vi "AlarmEngineBuildTags.vi"(8 "error in (no error)":errorcluster, 10 "Config":T2, 11 "ModuleID":string) -> (0 "error out":errorcluster, 3 "Tag Refs":T1)   [LabVIEW 2020, in "AlarmEngine.lvlib"]
uses:
  AlarmEngine.lvlib
  3621d97f-605c-4e6f-807d-a17beb1ed3ae.vi
  f8fd6500-b03e-4021-a7cb-1885c161f361.vi
  <vilib>/Tag Engine/Tag/Tag.lvclass
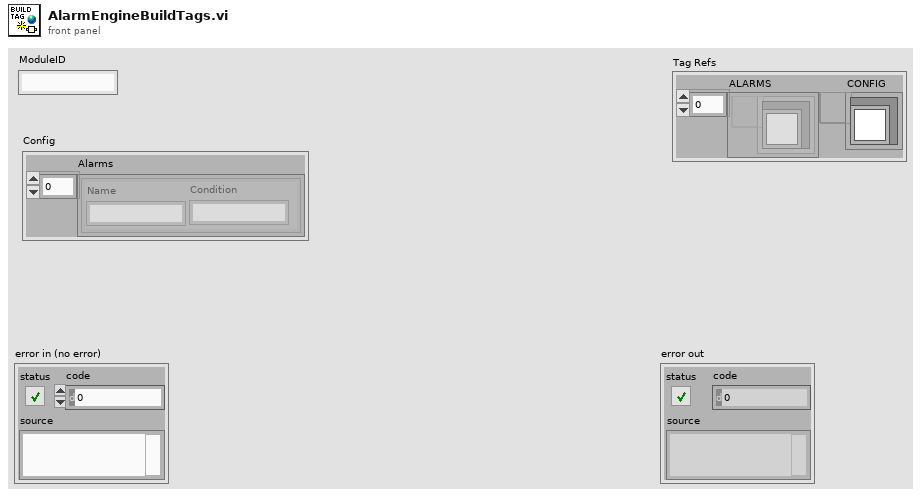
[diagram p1: front panel]
types:
  T1 = cluster{"ALARMS":refnum<data-value>[], "CONFIG":refnum<data-value>}
  T2 = cluster{"Alarms":cluster{"Name":string, "Condition":string}[]}
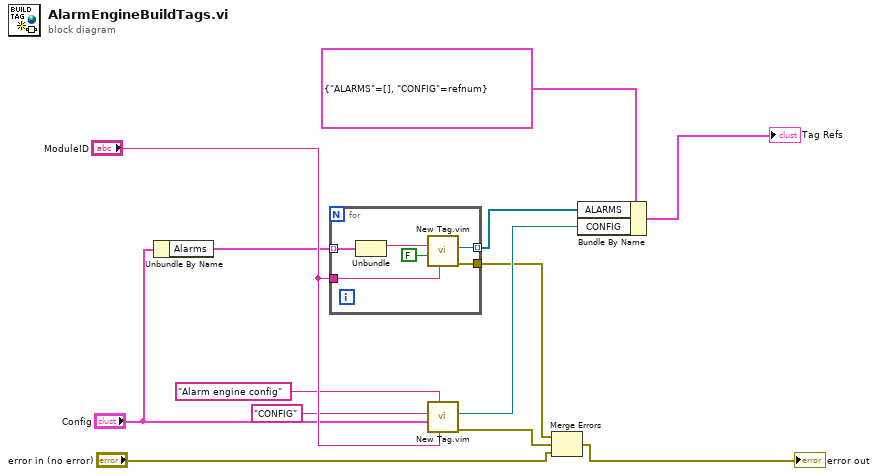
[diagram p0: block diagram]
diagram:
  n1 = Unbundle By Name("Config") -> ("Alarms"=w3:cluster{"Name":string, "Condition":string}[])
  n2 = for {
    tunnel: "ModuleID" -> [w19]
    tunnel: [w17] -> w10
    tunnel: w3 -> [w16] mode=indexing
    tunnel: [w14] -> w2 mode=indexing
    n3 = Unbundle(w16) -> ("Name"=w15:string)  [unwired: 1 out]
    n4 = call "New Tag.vim"("Namespace"=w19, "Initial Value"=FALSE, "Tag Name"=w15) -> ("error out"=w17:errorcluster, "Tag Ref out"=w14:refnum<data-value>)  [unwired: 7 in]
  }
  n5 = call "New Tag.vim"("Namespace"="ModuleID", "Description (none)"="Alarm engine config", "Initial Value"="Config", "Tag Name"="CONFIG") -> ("error out"=w9:errorcluster, "Tag Ref out"=w11:refnum<data-value>)  [unwired: 6 in]
  n6 = Merge Errors(w10, w9, "error in (no error)") -> (→"error out":errorcluster)
  n7 = Bundle By Name(cluster=T1 {"ALARMS"=[], "CONFIG"=refnum} ("Tag Refs"), "ALARMS"=w2, "CONFIG"=w11) -> (→"Tag Refs":T1)
